vi "Optitrack Position Server.vi"() -> (1 "Position XYZ":dbl[](array[numeric]) format="%.2f")   [LabVIEW 2022 SP3]
uses:
  Optitrack Global.vi
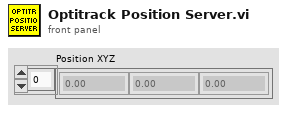
[diagram p1: front panel]
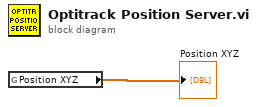
[diagram p0: block diagram]
diagram:
  n1 = global read "Optitrack Global.vi" "Position XYZ"() -> (→"Position XYZ":dbl[])
